vi "Host Troubleshoot Streams.vi"() -> ()   [LabVIEW 2018]
panel:
  out "error out":errorcluster
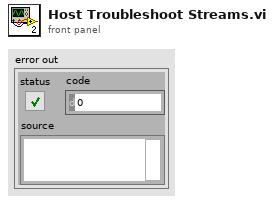
[diagram p1: front panel]
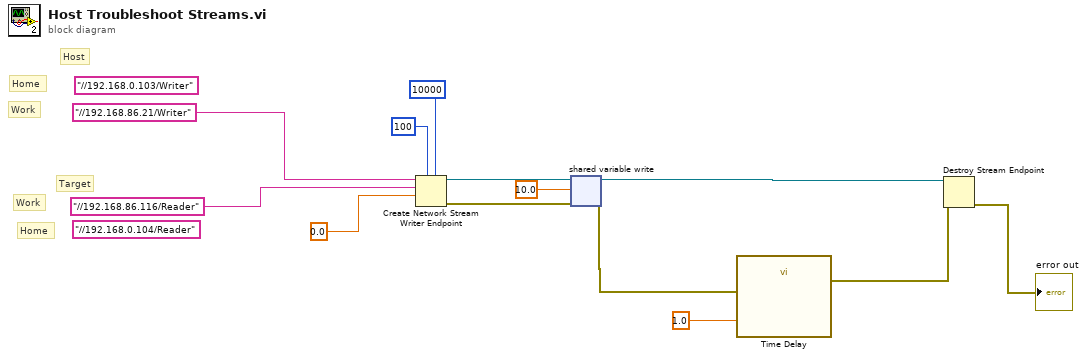
[diagram p0: block diagram]
diagram:
  (unwired) "//192.168.0.103/Writer" ("writer name")
  (unwired) "//192.168.0.104/Reader" ("reader url")
  # "Work"
  # "Work"
  # "Home"
  # "Home"
  # "Target"
  # "Host"
  n1 = Create Network Stream Writer Endpoint(5:10000 ("timeout in ms (-1)"), 7:100 ("writer buffer size"), 9:0.0, 10:"//192.168.86.116/Reader" ("reader url"), 11:"//192.168.86.21/Writer" ("writer name")) -> (0:w7:errorcluster, 3:w8:refnum<k21>)  [unwired: 2 in]
  n2 = shared-variable-write(w8, w7, 10.0 ("data in")) -> (w5:refnum<k21>, w3:errorcluster)  [unwired: 1 in, 1 out]
  n3 = call "Time Delay"("error in (no error)"=w3, "Delay Time (s)"=1.0) -> ("error out"=w2:errorcluster)  [unwired: 9 in]
  n4 = Destroy Stream Endpoint(8:w2, 11:w5) -> (0:→"error out":errorcluster)
